vi "BioFeedback10(SaveStabilityData).vi"(0 "UI Data Right":path=path "C:/Users/Tinggroup/Desktop/VRMuscleActivationVisualizer/VRBiofeedback_v2/assets/RightEMGData.txt", 7 "Frames Per Second":dbl=30.0, 9 "Start Trial":bool, 11 "End Trial":bool, 12 "Data Directory":path, 13 "File Name":string, 14 "Extension":string="_EMG.txt") -> ()   [LabVIEW 2016]
uses:
  <vilib>/Utility/error.llb/DialogType.ctl
  <vilib>/Analysis/5stat.llb/RMS (DBL).vi
  <vilib>/Waveform/WDTOps.llb/WDT Append Waveforms DBL.vi
  <vilib>/Waveform/WDTFileIO.llb/Export Waveforms To Spreadsheet File (1D).vi
  <vilib>/Analysis/NI_AALPro.lvlib
panel:
  out "ReturnData":dbl[](array[numeric])
  in  "StdDevIndex":dbl=3.0
  in  "MeanIndex":dbl=2.0
  in  "MaxIndex":dbl=1.0
  in  "MinIndex":dbl
  out "Stability Data":dbl[][](array[numeric])
  out "2d target":cluster{dbl[], dbl[]}[](graph)
  out "trialFilteredData":waveform(dbl)[](array[waveform])
  out "filteredWaveforms":waveform(dbl)[](array[waveform])
  in  "UI Ampl Error Path":path=path "C:/Users/Tinggroup/Desktop/VRMuscleActivationVisualizer/VRBiofeedback_v2/assets/BiofeedbackAmplitudeError.txt"
  in  "UI L/R Error Path":path=path "C:/Users/Tinggroup/Desktop/VRMuscleActivationVisualizer/VRBiofeedback_v2/assets/BiofeedbackLRError.txt"
  out "LeftPercentActivation":dbl
  out "RightPercentActivation":dbl
  out "LeftMovingAvg":dbl
  out "RightMovingAvg":dbl
  in  "AutoAnalyzeStablity":bool
  out "RMS Left Single Bucket":dbl(graph)
  out "PointCluster":cluster{dbl[], dbl[]}
  out "combined y value":dbl
  out "Acquiring Max":bool
  in  "endGetMax":bool
  in  "startGetMax":bool
  in  "Right Max":dbl
  in  "Left Max":dbl
  in  "Amplitude Error":dbl
  in  "L/R error":dbl
  in  "RightSignalB":dbl=6.0
  in  "RightSignalA":dbl=5.0
  in  "LefftSignalB":dbl=2.0
  in  "LeftSignalA":dbl=1.0
  out "Aggregate 8":waveform(dbl)[](array[waveform])
  in  "UI Data Left":path=path "C:/Users/Tinggroup/Desktop/VRMuscleActivationVisualizer/VRBiofeedback_v2/assets/LeftEMGData.txt"
  in  "EMG Input Device\nProduct Type":string="USB-6009"
  out "DispLeftMovingAvg":dbl(slide) caption="Left" max=1.0 scale=0.0..100.0
  out "DispRightMovingAvg":dbl(slide) caption="Right" max=0.01 scale=0.0..100.0
  out "RMS Right":dbl(graph)
  out "RMS Left":dbl(graph)
  out "RMS 8":dbl(graph)
  out "RMS 7":dbl(graph)
  out "RMS 6":dbl(graph)
  out "RMS 5":dbl(graph)
  out "RMS 4":dbl(graph)
  out "RMS 3":dbl(graph)
  out "RMS 2":dbl(graph)
  out "RMS 1":dbl(graph)
  out "Aggregate7":waveform(dbl)[](array[waveform])
  out "Aggregate6":waveform(dbl)[](array[waveform])
  out "Aggregate5":waveform(dbl)[](array[waveform])
  out "Aggregate4":waveform(dbl)[](array[waveform])
  out "Aggregate3":waveform(dbl)[](array[waveform])
  out "Aggregate2":waveform(dbl)[](array[waveform])
  out "Aggregate1":waveform(dbl)[](array[waveform])
  out "Wfm8":waveform(dbl)(graph)
  out "Wfm7":waveform(dbl)(graph)
  out "Wfm6":waveform(dbl)(graph)
  out "Wfm5":waveform(dbl)(graph)
  out "Wfm4":waveform(dbl)(graph)
  out "Wfm3":waveform(dbl)(graph)
  out "Wfm2":waveform(dbl)(graph)
  out "Wfm1":waveform(dbl)(graph)
  out "Trial Raw Waveforms":waveform(dbl)[](graph)
  in  "UI Percent Path":path=path "C:/Users/Tinggroup/Desktop/VRMuscleActivationVisualizer/VRBiofeedback_v2/assets/BiofeedbackTargetPercentage.txt"
  in  "Target Percentage":dbl=10.0
  out "Trial In Progress":bool
  in  "Lower Cut-Off":dbl=20.0
  in  "Upper Cut-Off":dbl=300.0
  out "raw data":dynamicdata(graph)
  out "Bufffer Index":dbl
  out "Frames in Buffer":dbl
  out "Samples per frame":dbl
  out "Reset Data Acquisition\nAnd UI Updating":bool=TRUE
  in  "Moving Average Length (s)":dbl=0.5
  in  "Sample rate (Hz)":dbl=2000.0
  in  "End Program":bool
  # "Saving Trial Data"
  # "Set Target and Box Size"
  # "Set Scale"
  # "These scale the thermometers and are used in mean calculation"
  # "Analyze Stability of Displayed Data"
  # "Auto Analyze Stability begins calculating stability\nAs soon as dot enters the target zone and stops \nonce the dot leaves the target zone (Not Yet Implemented)"
  # "Channels used in Display"
  # "Filter and Process Parameters"
  # "Dimension1 - Signal\nDimension2 - property"
  # "Min"
  # "Max"
  # "Mean"
  # "StdDev"
  # "Changes are made instantly and cause moving average to reset to zero"
  # "for testing smaller sample\nsizes in getting max/min\nand stability data"
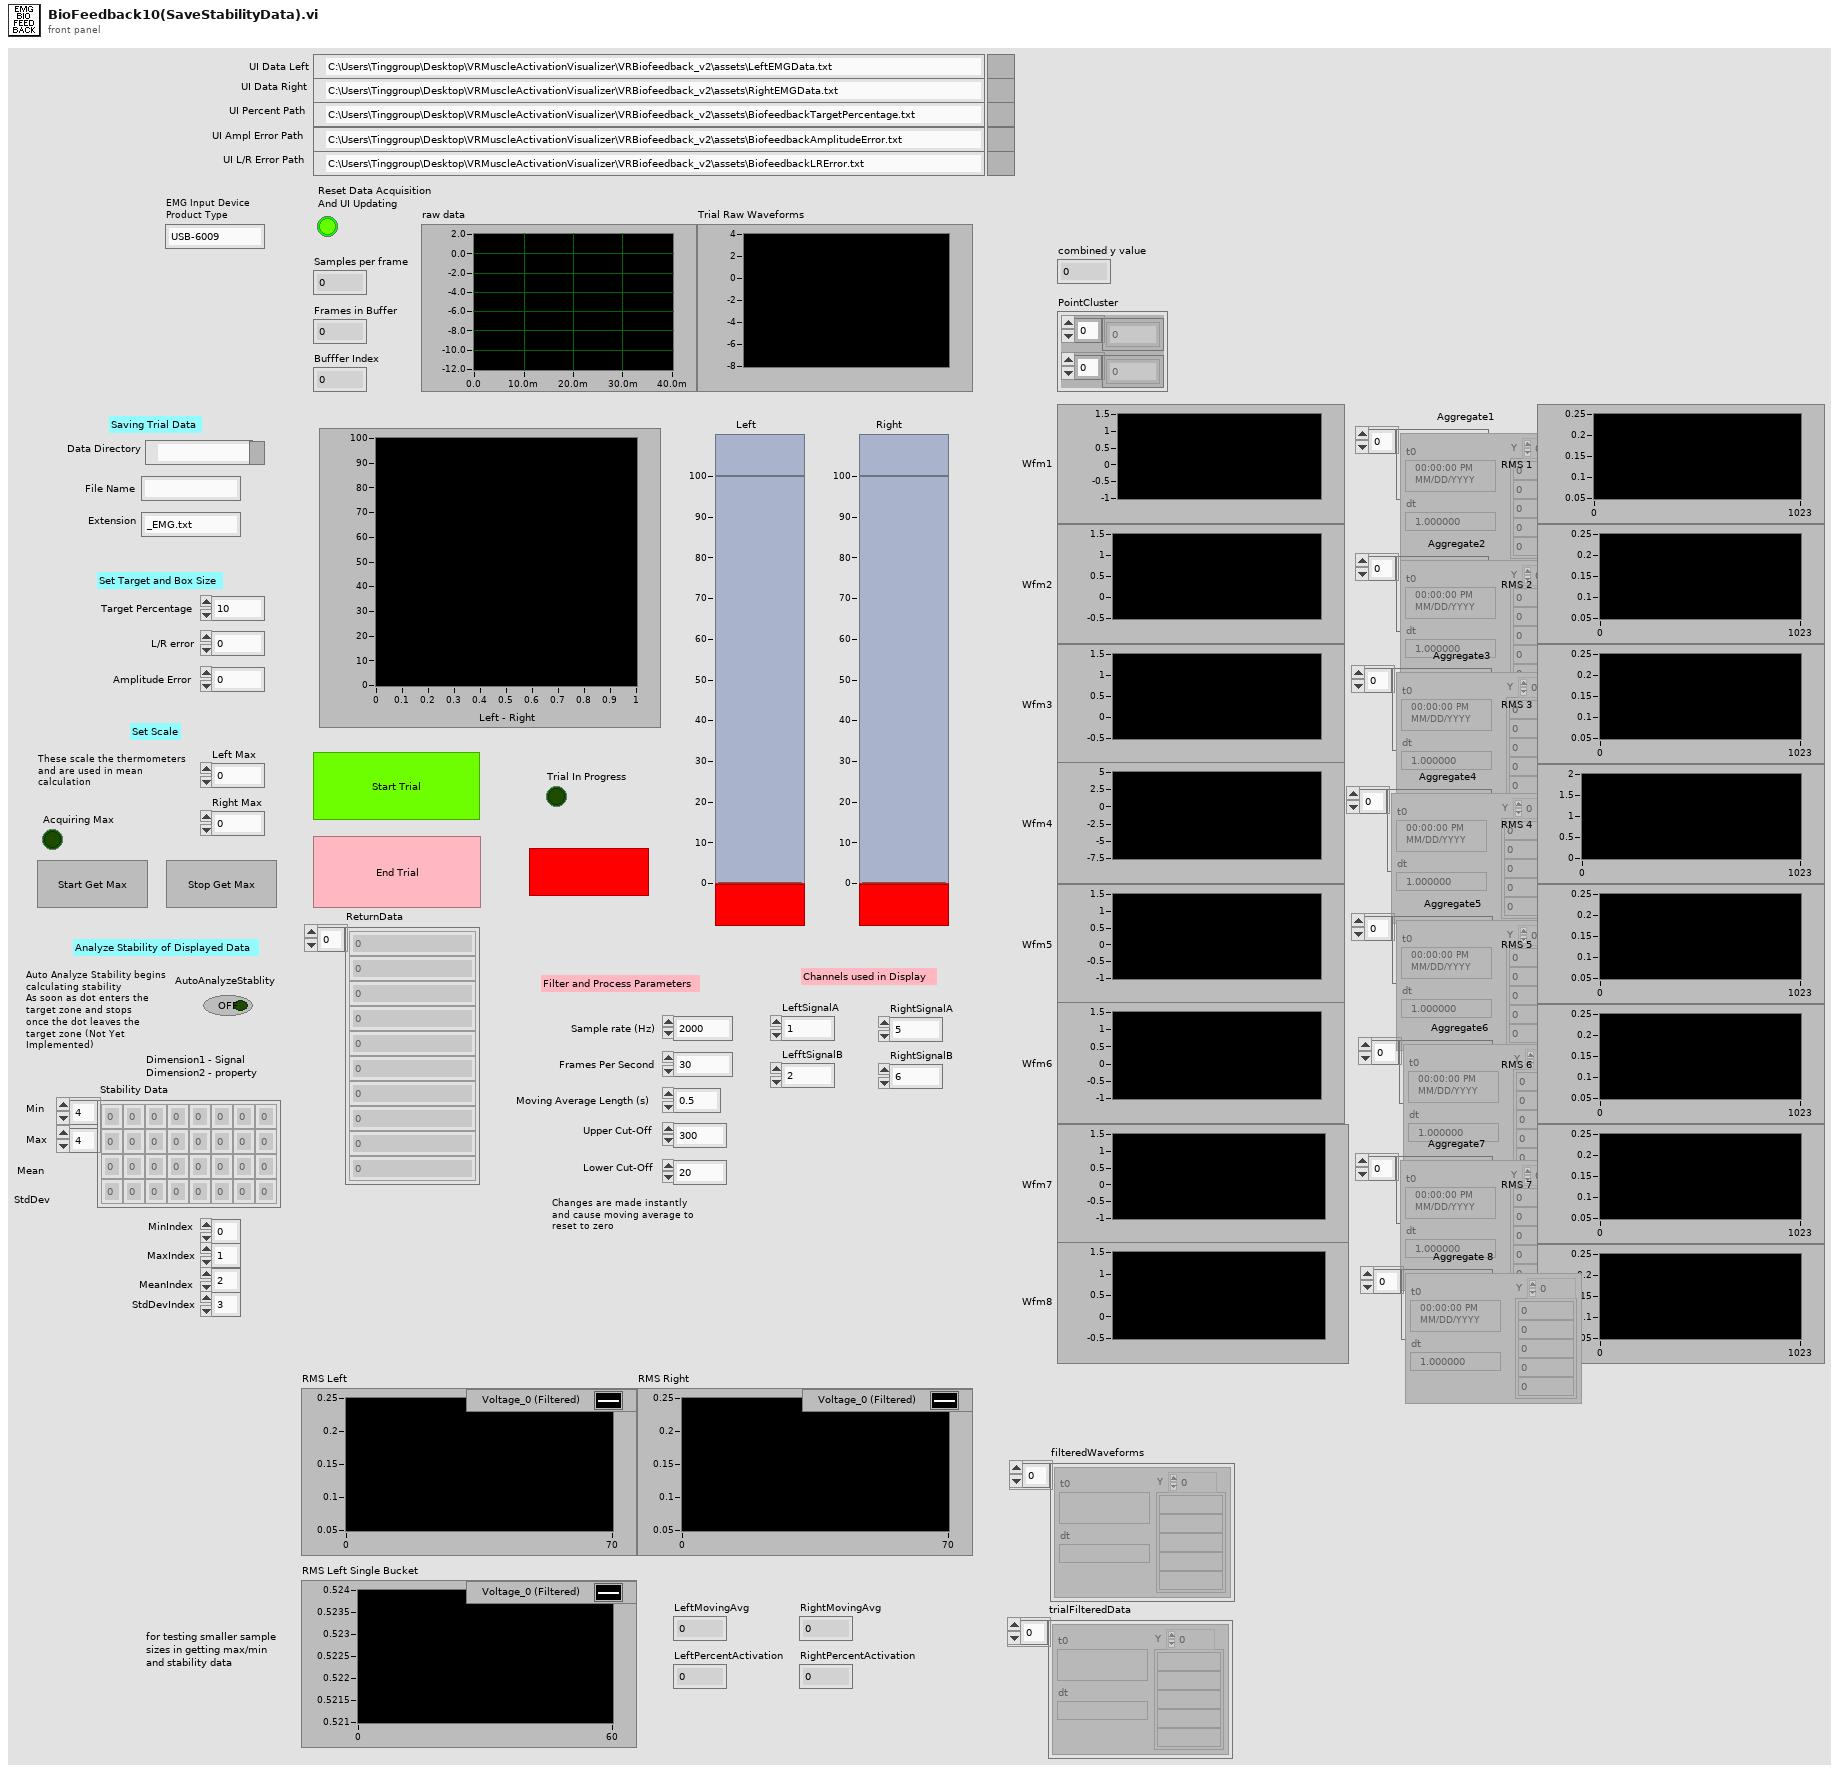
[diagram p1: front panel]
types:
  T1 = typedef "DialogType.ctl" = u16
  T2 = typedef "WaveformArrayControl.ctl" = waveform(dbl)[]
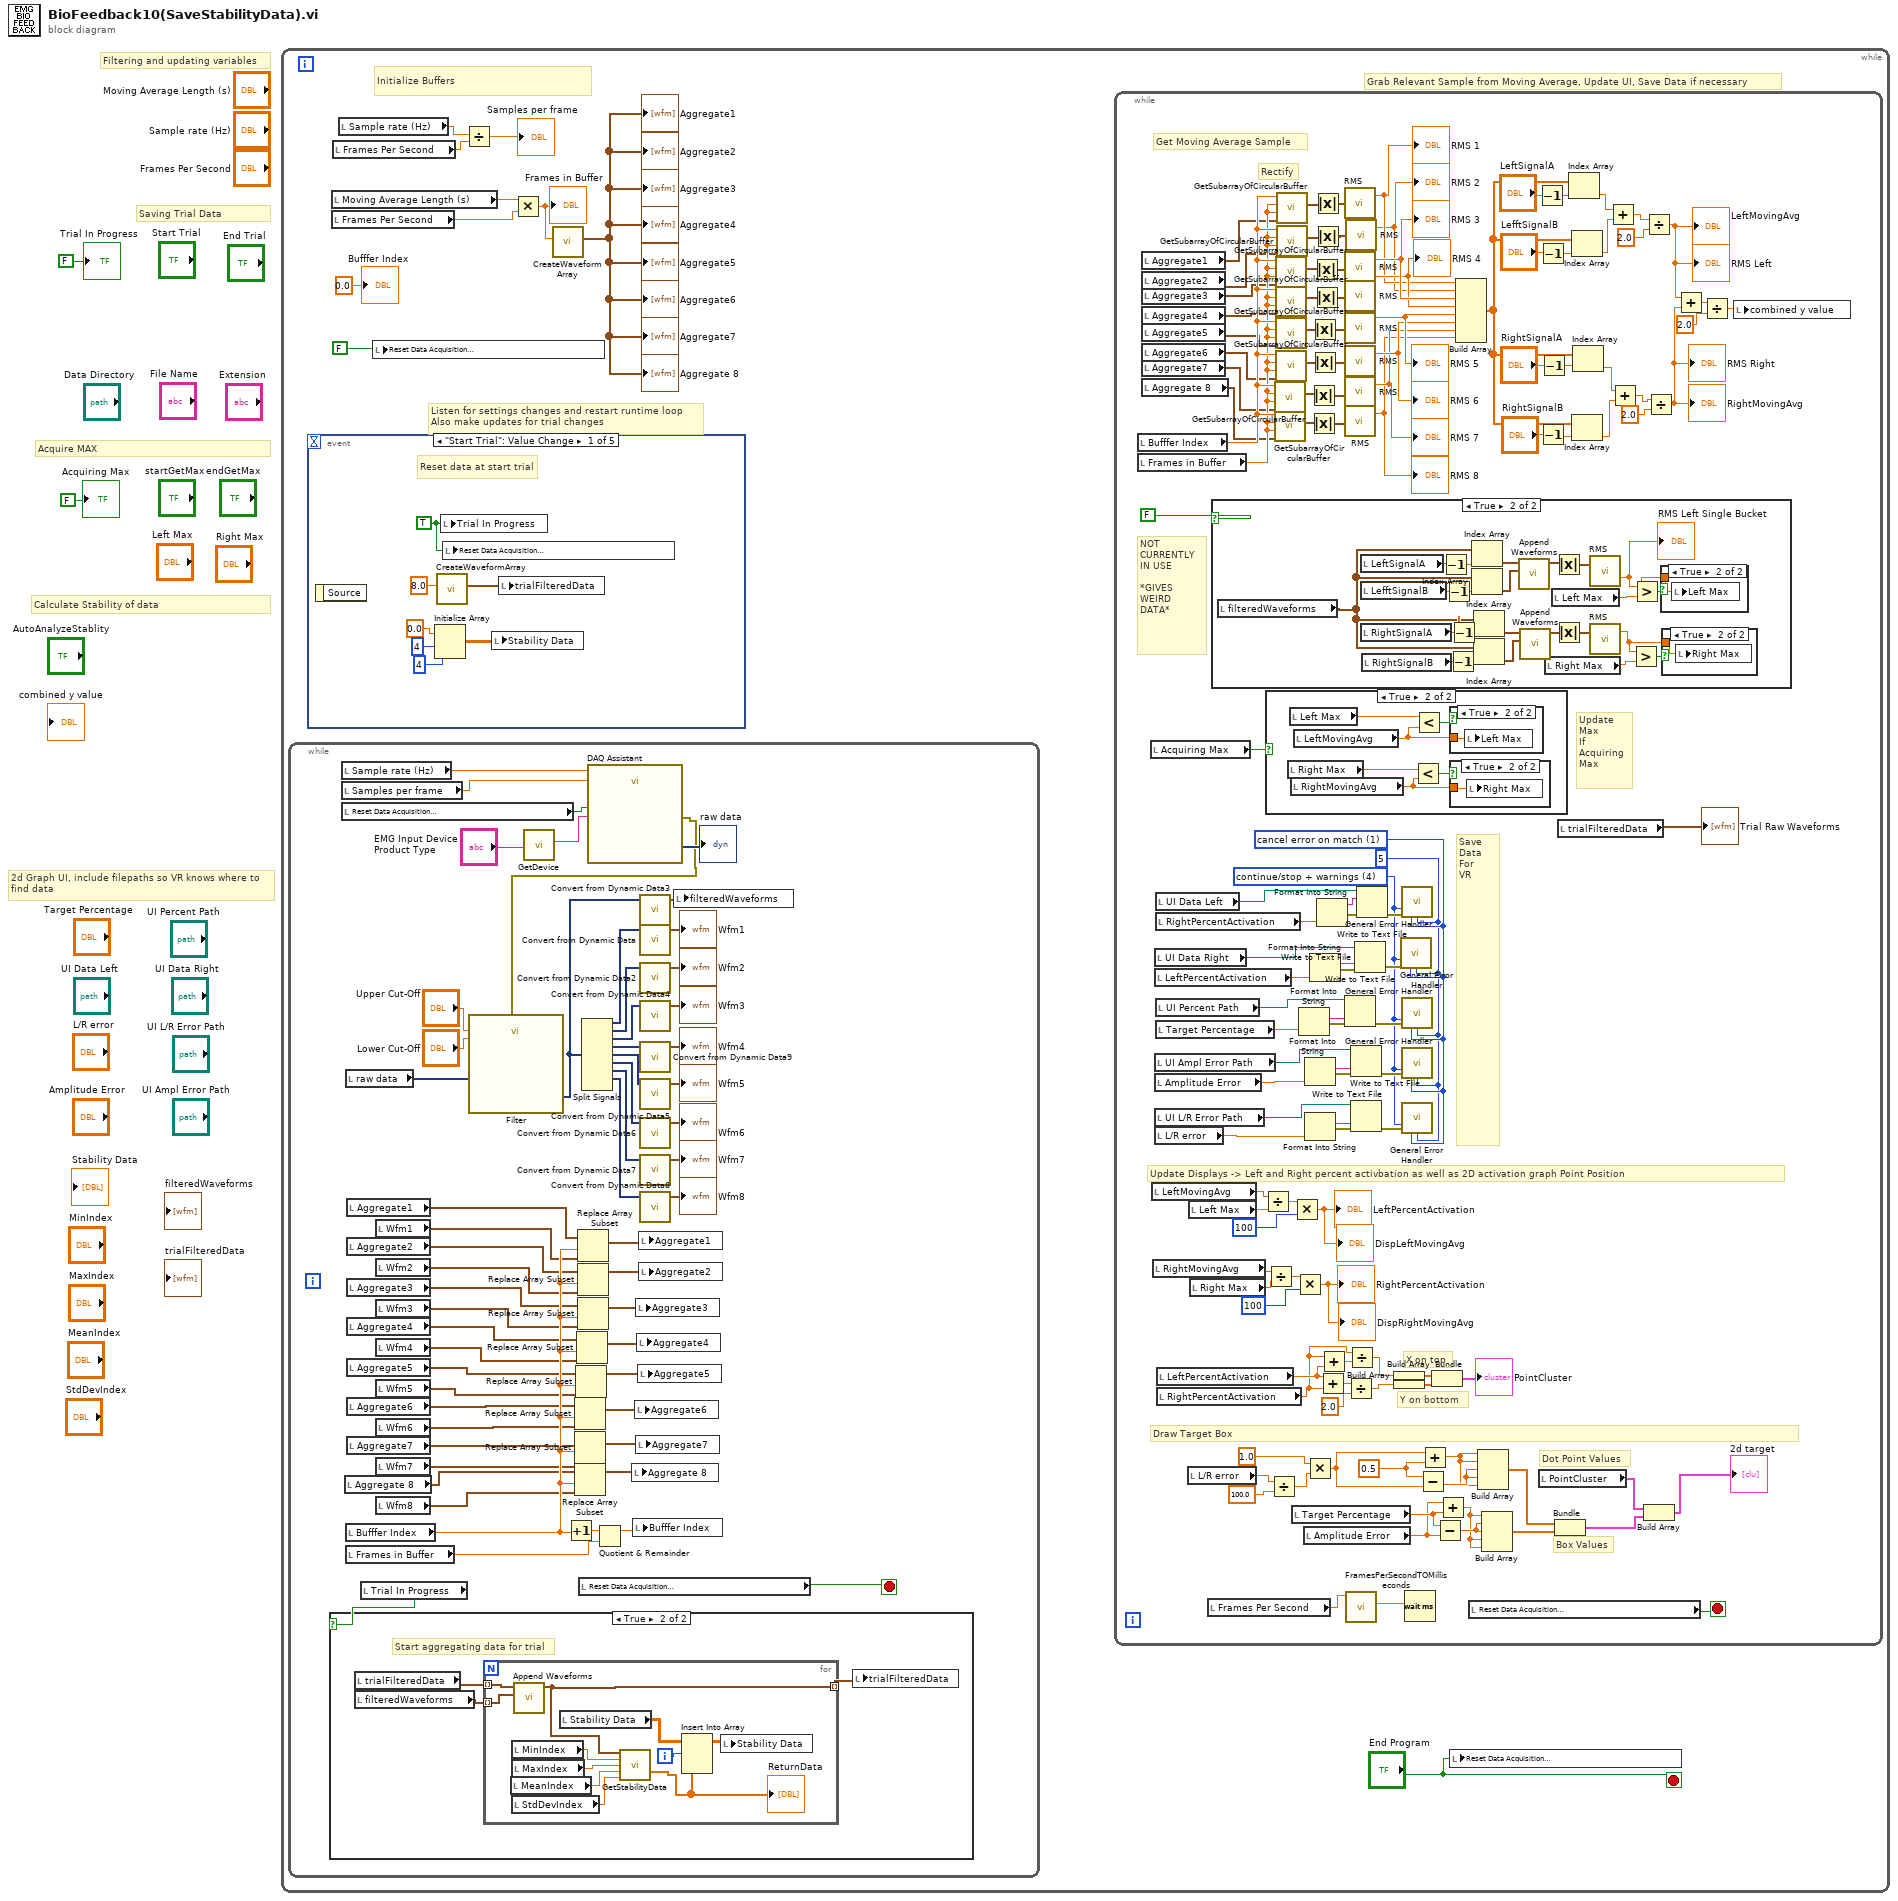
[diagram p0: block diagram]
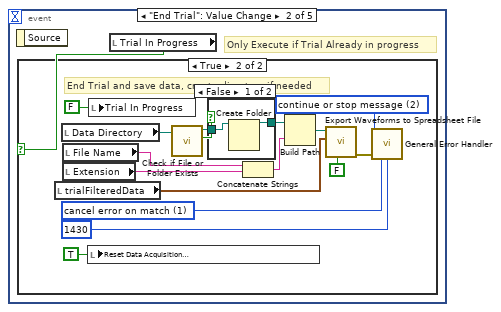
[diagram p2: hidden frame]
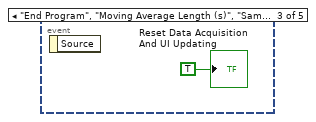
[diagram p5: hidden frame]
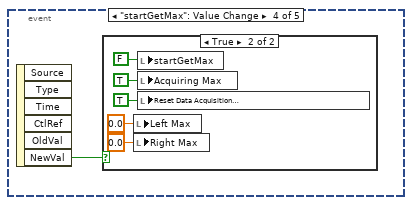
[diagram p6: hidden frame]
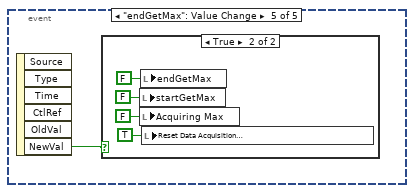
[diagram p8: hidden frame]
diagram:
  # "Calculate Stability of data"
  # "Acquire MAX"
  # "Filtering and updating variables"
  # "Saving Trial Data"
  # "2d Graph UI, include filepaths so VR knows where to find data"
  n1 = while {
    stop <- "End Program" stop-if-true
    # "Grab Relevant Sample from Moving Average, Update UI, Save Data if necessary"
    # "Initialize Buffers"
    # "Listen for settings changes and restart runtime loop\nAlso make updates for trial changes"
    n2 = while {
      stop <- w262 stop-if-true
      n3 = local read "Sample rate (Hz)"() -> (w269:dbl)
      n4 = local read "Samples per frame"() -> (w268:dbl)
      n5 = local read "Reset Data Acquisition\nAnd UI Updating"() -> (w261:bool)
      n6 = local read "Aggregate 8"() -> (w218:waveform(dbl)[])
      n7 = local read "raw data"() -> (w267:dynamicdata)
      n8 = local read "Bufffer Index"() -> (w243:dbl)
      n9 = local read "Frames in Buffer"() -> (w264:dbl)
      n10 = local read "Aggregate1"() -> (w242:waveform(dbl)[])
      n11 = local read "Aggregate2"() -> (w240:waveform(dbl)[])
      n12 = local read "Aggregate3"() -> (w238:waveform(dbl)[])
      n13 = local read "Aggregate4"() -> (w236:waveform(dbl)[])
      n14 = local read "Aggregate5"() -> (w234:waveform(dbl)[])
      n15 = local read "Aggregate6"() -> (w232:waveform(dbl)[])
      n16 = local read "Aggregate7"() -> (w230:waveform(dbl)[])
      n17 = local read "Trial In Progress"() -> (w220:bool)
      n18 = case shown="True" w220 {
        frame False {
        }
        frame True {
          # "Start aggregating data for trial"
          n19 = local read "trialFilteredData"() -> (w271:waveform(dbl)[])
          n20 = local read "filteredWaveforms"() -> (w272:waveform(dbl)[])
          n21 = for {
            tunnel: w272 -> [w282] mode=indexing
            tunnel: w271 -> [w283] mode=indexing
            tunnel: [w274] -> w270 mode=indexing
            i -> [w275]
            n22 = local read "MeanIndex"() -> (w278:dbl)
            n23 = local read "MinIndex"() -> (w276:dbl)
            n24 = local read "MaxIndex"() -> (w277:dbl)
            n25 = local read "StdDevIndex"() -> (w279:dbl)
            n26 = call-poly <vilib>:"Append Waveforms.vi"("waveform B"=w282, "waveform A"=w283) -> ("waveform out"=w274:waveform(dbl))  [unwired: 8 in, 1 out]
            n27 = local read "Stability Data"() -> (w280:dbl[][])
            n28 = call "GetStabilityData.vi"("ProvidedData"=w274, "MinIndex"=w276, "MaxIndex"=w277, "MeanIndex"=w278, "StdDevIndex"=w279) -> ("ReturnData"=w273:dbl[])  [unwired: 10 in]
            "ReturnData" <- w273
            n29 = Insert Into Array(array=w280, index (row)=w275, new element=w273) -> (w281:dbl[][])  [unwired: 1 in]
            n30 = local write "Stability Data"(w281) -> ()
          }
          n31 = local write "trialFilteredData"(w270) -> ()
        }
      }
      n32 = local read "Wfm1"() -> (w241:waveform(dbl))
      n33 = local read "Wfm2"() -> (w239:waveform(dbl))
      n34 = local read "Wfm3"() -> (w237:waveform(dbl))
      n35 = local read "Wfm4"() -> (w235:waveform(dbl))
      n36 = local read "Wfm5"() -> (w233:waveform(dbl))
      n37 = local read "Wfm6"() -> (w231:waveform(dbl))
      n38 = local read "Wfm7"() -> (w229:waveform(dbl))
      n39 = local read "Wfm8"() -> (w228:waveform(dbl))
      n40 = call "GetDevice.vi"("EMG Input Device\nProduct Type"="EMG Input Device\nProduct Type") -> ("DAQmx Device Name"=w216:tag)  [unwired: 10 in]
      n41 = Increment(x=w243) -> (x+1=w263:dbl)
      n42 = Replace Array Subset(array=w232, new element=w231, index=w243) -> (w222:waveform(dbl)[])
      n43 = Replace Array Subset(array=w230, new element=w229, index=w243) -> (w221:waveform(dbl)[])
      n44 = Replace Array Subset(array=w218, new element=w228, index=w243) -> (w219:waveform(dbl)[])
      n45 = Replace Array Subset(array=w234, new element=w233, index=w243) -> (w223:waveform(dbl)[])
      n46 = Replace Array Subset(array=w236, new element=w235, index=w243) -> (w224:waveform(dbl)[])
      n47 = Replace Array Subset(array=w242, new element=w241, index=w243) -> (w227:waveform(dbl)[])
      n48 = Replace Array Subset(array=w240, new element=w239, index=w243) -> (w226:waveform(dbl)[])
      n49 = Replace Array Subset(array=w238, new element=w237, index=w243) -> (w225:waveform(dbl)[])
      n50 = local read "Reset Data Acquisition\nAnd UI Updating"() -> (w262:bool)
      n51 = call "DAQ Assistant"("rate"=w269, "number of samples"=w268, "stop (T)"=w261, "device name"=w216) -> ("data"=→"raw data":dynamicdata, "error out"=w213:errorcluster)  [unwired: 13 in, 1 out]
      n52 = call "Filter"("error in (no error)"=w213, "Lower Cut-Off"="Lower Cut-Off", "Upper Cut-Off"="Upper Cut-Off", "Signal"=w267) -> ("Filtered Signal"=w212:dynamicdata)  [unwired: 6 in, 1 out]
      n53 = Split Signals(w212) -> (w259:dynamicdata, w258:dynamicdata, w257:dynamicdata, w256:dynamicdata, w255:dynamicdata, w254:dynamicdata, w253:dynamicdata, w252:dynamicdata)  [unwired: 9 in, 1 out]
      n54 = Quotient & Remainder(x=w263, y=w264) -> (x-y*floor(x/y)=w265:dbl)  [unwired: 1 out]
      n55 = local write "Aggregate 8"(w219) -> ()
      n56 = local write "Bufffer Index"(w265) -> ()
      n57 = local write "Aggregate6"(w222) -> ()
      n58 = local write "Aggregate3"(w225) -> ()
      n59 = local write "Aggregate7"(w221) -> ()
      n60 = local write "Aggregate4"(w224) -> ()
      n61 = local write "Aggregate5"(w223) -> ()
      n62 = local write "Aggregate1"(w227) -> ()
      n63 = local write "Aggregate2"(w226) -> ()
      n64 = call "Convert from Dynamic Data3"("Dynamic Data Type"=w212) -> ("Array of Waveform"=w214:waveform(dbl)[])  [unwired: 3 in]
      n65 = call "Convert from Dynamic Data"("Dynamic Data Type"=w259) -> ("Waveform"=→"Wfm1":waveform(dbl))  [unwired: 3 in]
      n66 = call "Convert from Dynamic Data2"("Dynamic Data Type"=w258) -> ("Waveform"=→"Wfm2":waveform(dbl))  [unwired: 3 in]
      n67 = call "Convert from Dynamic Data4"("Dynamic Data Type"=w257) -> ("Waveform"=→"Wfm3":waveform(dbl))  [unwired: 3 in]
      n68 = call "Convert from Dynamic Data9"("Dynamic Data Type"=w256) -> ("Waveform"=→"Wfm4":waveform(dbl))  [unwired: 3 in]
      n69 = call "Convert from Dynamic Data5"("Dynamic Data Type"=w255) -> ("Waveform"=→"Wfm5":waveform(dbl))  [unwired: 3 in]
      n70 = call "Convert from Dynamic Data6"("Dynamic Data Type"=w254) -> ("Waveform"=→"Wfm6":waveform(dbl))  [unwired: 3 in]
      n71 = call "Convert from Dynamic Data7"("Dynamic Data Type"=w253) -> ("Waveform"=→"Wfm7":waveform(dbl))  [unwired: 3 in]
      n72 = call "Convert from Dynamic Data8"("Dynamic Data Type"=w252) -> ("Waveform"=→"Wfm8":waveform(dbl))  [unwired: 3 in]
      n73 = local write "filteredWaveforms"(w214) -> ()
    }
    n74 = event shown="[0] \"Start Trial\": Value Change" {
      selector: _ -> [_ _ _ _ _]
      dyn-events: _ -> [_ _ _ _ _]
      timeout: _ -> [_ _ _ _ _]
      event "Start Trial": Value Change {
        w19 = TRUE ("Trial In Progress")
        # "Reset data at start trial"
        n75 = event-data() -> ()  [unwired: 1 in, 1 out]
        n76 = Initialize Array(0.0 ("element"), 4 ("dimension size"), 4 ("dimension size")) -> (w13:dbl[][])
        n77 = call "CreateWaveformArray.vi"("bufferSize"=8.0) -> ("initialized array"=w18:waveform(dbl)[])  [unwired: 5 in, 1 out]
        n78 = local write "Trial In Progress"(w19) -> ()
        n79 = local write "Reset Data Acquisition\nAnd UI Updating"(w19) -> ()
        n80 = local write "Stability Data"(w13) -> ()
        n81 = local write "trialFilteredData"(w18) -> ()
      }
      event "End Trial": Value Change {
        # "Only Execute if Trial Already in progress"
        n82 = event-data() -> ()  [unwired: 1 in, 1 out]
        n83 = local read "Trial In Progress"() -> (w20:bool)
        n84 = case shown="True" w20 {
          frame False {
          }
          frame True {
            w29 = T1 2 items=["no dialog", "OK message", "continue or stop message", "OK message + warnings", "continue/stop + warnings"] ("type of dialog (OK msg:1)")
            w30 = 1 items=["no exception", "cancel error on match", "set error on match"] ("[exception action] (none:0)")
            # "End Trial and save data, create directory if needed"
            n85 = local read "trialFilteredData"() -> (w22:waveform(dbl)[])
            n86 = local read "Data Directory"() -> (w32:path)
            n87 = local read "File Name"() -> (w24:string)
            n88 = local read "Extension"() -> (w25:string)
            n89 = local write "Reset Data Acquisition\nAnd UI Updating"(TRUE ("Reset Data Acquisition\nAnd UI Updating")) -> ()
            n90 = local write "Trial In Progress"(FALSE ("Trial In Progress")) -> ()
            n91 = call <vilib>:"Check if File or Folder Exists.vi"("path"=w32) -> ("file or folder exists?"=w34:bool, "dup path"=w33:path)  [unwired: 8 in, 1 out]
            n92 = case shown="False" w34 {
              tunnel: [w37 w39] -> w28
              tunnel: w33 -> [w38 w39]
              frame False {
                n93 = Create Folder(path (use dialog)=w38) -> (created path=w37:path)  [unwired: 2 in, 2 out]
              }
              frame True {
              }
            }
            n94 = Concatenate Strings(w24, w25) -> (w23:string)
            n95 = Build Path(base path=w28, name or relative path=w23) -> (appended path=w27:path)
            n96 = call-poly <vilib>:"Export Waveforms to Spreadsheet File.vi"("append to file? (new file:F)"=FALSE, "waveforms"=w22, "file path (dialog if empty)"=w27) -> ("error out"=w21:errorcluster)  [unwired: 7 in, 1 out]
            n97 = call <vilib>:"General Error Handler.vi"("type of dialog (OK msg:1)"=w29, "error in (no error)"=w21, "[exception action] (none:0)"=w30, "[exception code]"=1430) -> ()  [unwired: 7 in, 5 out]
          }
        }
      }
      event "End Program", "Moving Average Length (s)", "Sample rate (Hz)", "Frames Per Second": Value Change {
        n98 = event-data() -> ()  [unwired: 1 in, 1 out]
        "Reset Data Acquisition\nAnd UI Updating" <- TRUE
      }
      event "startGetMax": Value Change {
        n99 = event-data() -> ("NewVal"=w41:bool)  [unwired: 1 in, 5 out]
        n100 = case shown="True" w41 {
          frame False {
          }
          frame True {
            n101 = local write "Left Max"(0.0 ("Left Max")) -> ()
            n102 = local write "Right Max"(0.0 ("Right Max")) -> ()
            n103 = local write "startGetMax"(FALSE) -> ()
            n104 = local write "Acquiring Max"(TRUE ("Acquiring Max")) -> ()
            n105 = local write "Reset Data Acquisition\nAnd UI Updating"(TRUE ("Reset Data Acquisition\nAnd UI Updating")) -> ()
          }
        }
      }
      event "endGetMax": Value Change {
        n106 = event-data() -> ("NewVal"=w47:bool)  [unwired: 1 in, 5 out]
        n107 = case shown="True" w47 {
          frame False {
          }
          frame True {
            n108 = local write "startGetMax"(FALSE ("startGetMax")) -> ()
            n109 = local write "Acquiring Max"(FALSE ("Acquiring Max")) -> ()
            n110 = local write "endGetMax"(FALSE ("endGetMax")) -> ()
            n111 = local write "Reset Data Acquisition\nAnd UI Updating"(TRUE ("Reset Data Acquisition\nAnd UI Updating")) -> ()
          }
        }
      }
    }
    n112 = local read "Moving Average Length (s)"() -> (w9:dbl)
    n113 = local read "Frames Per Second"() -> (w8:dbl)
    n114 = local read "Frames Per Second"() -> (w11:dbl)
    n115 = local read "Sample rate (Hz)"() -> (w12:dbl)
    n116 = local write "Reset Data Acquisition\nAnd UI Updating"(FALSE) -> ()
    n117 = Divide(x=w12, y=w11) -> (x/y=→"Samples per frame":dbl)
    n118 = Multiply(x=w9, y=w8) -> (x*y=w5:dbl)
    "Frames in Buffer" <- w5
    n119 = call "CreateWaveformArray.vi"("bufferSize"=w5) -> ("initialized array"=→"Aggregate1" →"Aggregate2" →"Aggregate3" →"Aggregate4" →"Aggregate5" →"Aggregate6" →"Aggregate7" →"Aggregate 8":waveform(dbl)[])  [unwired: 5 in, 1 out]
    n120 = while {
      stop <- w178 stop-if-true
      w104 = 0.5 ("element")
      w57 = T1 4 items=["no dialog", "OK message", "continue or stop message", "OK message + warnings", "continue/stop + warnings"] ("type of dialog (OK msg:1)")
      w56 = 1 items=["no exception", "cancel error on match", "set error on match"] ("[exception action] (none:0)")
      w55 = 5 ("[exception code]")
      # "Y on bottom"
      # "X on top"
      # "Dot Point Values"
      # "Box Values"
      # "Update Displays -> Left and Right percent activbation as well as 2D activation graph Point Position"
      # "NOT\nCURRENTLY\nIN USE\n\n*GIVES\nWEIRD\nDATA*"
      # "Draw Target Box"
      # "Update\nMax\nIf \nAcquiring\nMax"
      # "Save\nData\nFor\nVR"
      # "Get Moving Average Sample"
      # "Rectify"
      n121 = local read "Bufffer Index"() -> (w169:dbl)
      n122 = local read "Frames in Buffer"() -> (w168:dbl)
      n123 = local read "Aggregate1"() -> (w167:waveform(dbl)[])
      n124 = local read "Aggregate2"() -> (w163:waveform(dbl)[])
      n125 = local read "Aggregate3"() -> (w166:waveform(dbl)[])
      n126 = local read "Aggregate4"() -> (w162:waveform(dbl)[])
      n127 = local read "Aggregate5"() -> (w165:waveform(dbl)[])
      n128 = local read "Aggregate6"() -> (w164:waveform(dbl)[])
      n129 = local read "Aggregate7"() -> (w161:waveform(dbl)[])
      n130 = local read "Aggregate 8"() -> (w135:waveform(dbl)[])
      n131 = local read "Acquiring Max"() -> (w90:bool)
      n132 = local read "LeftMovingAvg"() -> (w86:dbl)
      n133 = local read "RightMovingAvg"() -> (w82:dbl)
      n134 = local read "UI Data Right"() -> (w173:path)
      n135 = local read "LeftPercentActivation"() -> (w171:dbl)
      n136 = local read "UI Ampl Error Path"() -> (w58:path)
      n137 = local read "Amplitude Error"() -> (w59:dbl)
      n138 = local read "UI L/R Error Path"() -> (w61:path)
      n139 = local read "L/R error"() -> (w60:dbl)
      n140 = local read "UI Data Left"() -> (w143:path)
      n141 = local read "RightPercentActivation"() -> (w145:dbl)
      n142 = local read "UI Percent Path"() -> (w137:path)
      n143 = local read "Target Percentage"() -> (w136:dbl)
      n144 = local read "LeftPercentActivation"() -> (w75:dbl)
      n145 = local read "RightPercentActivation"() -> (w73:dbl)
      n146 = local read "L/R error"() -> (w115:dbl)
      n147 = local read "Left Max"() -> (w85:dbl)
      n148 = local read "Right Max"() -> (w81:dbl)
      n149 = local read "Frames Per Second"() -> (w177:dbl)
      n150 = case shown="True" FALSE {
        frame False {
        }
        frame True {
          n151 = local read "filteredWaveforms"() -> (w187:waveform(dbl)[])
          n152 = local read "LeftSignalA"() -> (w195:dbl)
          n153 = local read "LefftSignalB"() -> (w193:dbl)
          n154 = local read "RightSignalA"() -> (w191:dbl)
          n155 = local read "RightSignalB"() -> (w188:dbl)
          n156 = Decrement(x=w195) -> (x-1=w194:dbl)
          n157 = Decrement(x=w193) -> (x-1=w192:dbl)
          n158 = Decrement(x=w188) -> (x-1=w189:dbl)
          n159 = Decrement(x=w191) -> (x-1=w190:dbl)
          n160 = Index Array(array=w187, index=w194) -> (element=w196:waveform(dbl))
          n161 = Index Array(array=w187, index=w192) -> (element=w197:waveform(dbl))
          n162 = Index Array(array=w187, index=w190) -> (element=w208:waveform(dbl))
          n163 = Index Array(array=w187, index=w189) -> (element=w207:waveform(dbl))
          n164 = call-poly <vilib>:"Append Waveforms.vi"("waveform B"=w197, "waveform A"=w196) -> ("waveform out"=w203:waveform(dbl))  [unwired: 8 in, 1 out]
          n165 = call-poly <vilib>:"Append Waveforms.vi"("waveform B"=w207, "waveform A"=w208) -> ("waveform out"=w206:waveform(dbl))  [unwired: 8 in, 1 out]
          n166 = local read "Right Max"() -> (w202:dbl)
          n167 = local read "Left Max"() -> (w209:dbl)
          n168 = Absolute Value(x=w203) -> (abs(x)=w204:waveform(dbl))
          n169 = Absolute Value(x=w206) -> (abs(x)=w205:waveform(dbl))
          n170 = call-poly <vilib>:"RMS.vi"("X"=w204) -> ("rms value"=w198:dbl)  [unwired: 1 out]
          "RMS Left Single Bucket" <- w198
          n171 = call-poly <vilib>:"RMS.vi"("X"=w205) -> ("rms value"=w201:dbl)  [unwired: 1 out]
          n172 = Greater?(x=w201, y=w202) -> (0:w200:bool)
          n173 = Greater?(x=w198, y=w209) -> (0:w199:bool)
          n174 = case shown="True" w199 {
            tunnel: w198 -> [_ w211]
            frame False {
            }
            frame True {
              n175 = local write "Left Max"(w211) -> ()
            }
          }
          n176 = case shown="True" w200 {
            tunnel: w201 -> [_ w210]
            frame False {
            }
            frame True {
              n177 = local write "Right Max"(w210) -> ()
            }
          }
        }
      }
      n178 = Divide(x=w86, y=w85) -> (x/y=w87:dbl)
      n179 = case shown="True" w90 {
        frame False {
        }
        frame True {
          n180 = local read "Right Max"() -> (w181:dbl)
          n181 = local read "Left Max"() -> (w184:dbl)
          n182 = local read "RightMovingAvg"() -> (w179:dbl)
          n183 = local read "LeftMovingAvg"() -> (w183:dbl)
          n184 = Less?(x=w181, y=w179) -> (x < y?=w180:bool)
          n185 = Less?(x=w184, y=w183) -> (x < y?=w182:bool)
          n186 = case shown="True" w182 {
            tunnel: w183 -> [_ w186]
            frame False {
            }
            frame True {
              n187 = local write "Left Max"(w186) -> ()
            }
          }
          n188 = case shown="True" w180 {
            tunnel: w179 -> [_ w185]
            frame False {
            }
            frame True {
              n189 = local write "Right Max"(w185) -> ()
            }
          }
        }
      }
      n190 = Divide(x=w82, y=w81) -> (x/y=w83:dbl)
      n191 = Divide(x=w115, y=100.0) -> (x/y=w109:dbl)
      n192 = call "GetSubarrayOfCircularBuffer.vi"("initialized array"=w161, "buffer size"=w168, "subset size"=w168, "start index"=w169) -> ("initialized array 2"=w154:T2)  [unwired: 7 in]
      n193 = call "GetSubarrayOfCircularBuffer.vi"("initialized array"=w135, "buffer size"=w168, "subset size"=w168, "start index"=w169) -> ("initialized array 2"=w153:T2)  [unwired: 7 in]
      n194 = call "GetSubarrayOfCircularBuffer.vi"("initialized array"=w166, "buffer size"=w168, "subset size"=w168, "start index"=w169) -> ("initialized array 2"=w158:T2)  [unwired: 7 in]
      n195 = call "GetSubarrayOfCircularBuffer.vi"("initialized array"=w162, "buffer size"=w168, "subset size"=w168, "start index"=w169) -> ("initialized array 2"=w157:T2)  [unwired: 7 in]
      n196 = call "GetSubarrayOfCircularBuffer.vi"("initialized array"=w165, "buffer size"=w168, "subset size"=w168, "start index"=w169) -> ("initialized array 2"=w156:T2)  [unwired: 7 in]
      n197 = call "GetSubarrayOfCircularBuffer.vi"("initialized array"=w164, "buffer size"=w168, "subset size"=w168, "start index"=w169) -> ("initialized array 2"=w155:T2)  [unwired: 7 in]
      n198 = call "GetSubarrayOfCircularBuffer.vi"("initialized array"=w167, "buffer size"=w168, "subset size"=w168, "start index"=w169) -> ("initialized array 2"=w160:T2)  [unwired: 7 in]
      n199 = call "GetSubarrayOfCircularBuffer.vi"("initialized array"=w163, "buffer size"=w168, "subset size"=w168, "start index"=w169) -> ("initialized array 2"=w159:T2)  [unwired: 7 in]
      n200 = Multiply(x=w87, y=100) -> (x*y=→"DispLeftMovingAvg" →"LeftPercentActivation":dbl)
      n201 = local read "Target Percentage"() -> (w54:dbl)
      n202 = Multiply(x=w83, y=100) -> (x*y=→"DispRightMovingAvg" →"RightPercentActivation":dbl)
      n203 = Format Into String(w136) -> (resulting string=w138:string, error out=w139:errorcluster)  [unwired: 3 in]
      n204 = local read "Amplitude Error"() -> (w53:dbl)
      n205 = Format Into String(w59) -> (resulting string=w65:string, error out=w66:errorcluster)  [unwired: 3 in]
      n206 = Format Into String(w60) -> (resulting string=w62:string, error out=w63:errorcluster)  [unwired: 3 in]
      n207 = Multiply(x=1.0, y=w109) -> (x*y=w108:dbl)
      n208 = Absolute Value(x=w154) -> (abs(x)=w147:T2)
      n209 = Absolute Value(x=w153) -> (abs(x)=w146:T2)
      n210 = Absolute Value(x=w156) -> (abs(x)=w149:T2)
      n211 = Absolute Value(x=w155) -> (abs(x)=w148:T2)
      n212 = Format Into String(w171) -> (resulting string=w172:string, error out=w174:errorcluster)  [unwired: 3 in]
      n213 = Absolute Value(x=w158) -> (abs(x)=w151:T2)
      n214 = Absolute Value(x=w157) -> (abs(x)=w150:T2)
      n215 = Absolute Value(x=w160) -> (abs(x)=w152:T2)
      n216 = Absolute Value(x=w159) -> (abs(x)=w134:T2)
      n217 = Format Into String(w145) -> (resulting string=w142:string, error out=w144:errorcluster)  [unwired: 3 in]
      n218 = Add(x=w75, y=w73) -> (x+y=w77:dbl)
      n219 = Add(x=w73, y=w75) -> (x+y=w74:dbl)
      n220 = call-poly <vilib>:"RMS.vi"("X"=w152) -> ("rms value"=w128:dbl)  [unwired: 1 out]
      "RMS 1" <- w128
      n221 = call-poly <vilib>:"RMS.vi"("X"=w151) -> ("rms value"=w133:dbl)  [unwired: 1 out]
      "RMS 3" <- w133
      n222 = call-poly <vilib>:"RMS.vi"("X"=w150) -> ("rms value"=w132:dbl)  [unwired: 1 out]
      "RMS 4" <- w132
      n223 = call-poly <vilib>:"RMS.vi"("X"=w149) -> ("rms value"=w131:dbl)  [unwired: 1 out]
      "RMS 5" <- w131
      n224 = call-poly <vilib>:"RMS.vi"("X"=w148) -> ("rms value"=w130:dbl)  [unwired: 1 out]
      "RMS 6" <- w130
      n225 = call-poly <vilib>:"RMS.vi"("X"=w147) -> ("rms value"=w129:dbl)  [unwired: 1 out]
      "RMS 7" <- w129
      n226 = call-poly <vilib>:"RMS.vi"("X"=w146) -> ("rms value"=w126:dbl)  [unwired: 1 out]
      "RMS 8" <- w126
      n227 = Write to Text File(file (use dialog)=w137, text=w138, error in=w139) -> (error out=w140:errorcluster)  [unwired: 1 in, 2 out]
      n228 = call-poly <vilib>:"RMS.vi"("X"=w134) -> ("rms value"=w127:dbl)  [unwired: 1 out]
      "RMS 2" <- w127
      n229 = Divide(x=w77, y=2.0) -> (x/y=w76:dbl)
      n230 = call "FramesPerSecondTOMilliseconds.vi"("Thermometer\nFps"=w177) -> ("x*y"=w176:dbl)  [unwired: 10 in]
      n231 = Divide(x=w73, y=w74) -> (x/y=w72:dbl)
      n232 = Write to Text File(file (use dialog)=w58, text=w65, error in=w66) -> (error out=w67:errorcluster)  [unwired: 1 in, 2 out]
      n233 = Write to Text File(file (use dialog)=w61, text=w62, error in=w63) -> (error out=w64:errorcluster)  [unwired: 1 in, 2 out]
      n234 = Write to Text File(file (use dialog)=w173, text=w172, error in=w174) -> (error out=w175:errorcluster)  [unwired: 1 in, 2 out]
      n235 = Write to Text File(file (use dialog)=w143, text=w142, error in=w144) -> (error out=w141:errorcluster)  [unwired: 1 in, 2 out]
      n236 = Build Array(w72) -> (w120:dbl[])
      n237 = Build Array(w76) -> (w118:dbl[])
      n238 = call <vilib>:"General Error Handler.vi"("type of dialog (OK msg:1)"=w57, "error in (no error)"=w175, "[exception action] (none:0)"=w56, "[exception code]"=w55) -> ()  [unwired: 7 in, 5 out]
      n239 = call <vilib>:"General Error Handler.vi"("type of dialog (OK msg:1)"=w57, "error in (no error)"=w141, "[exception action] (none:0)"=w56, "[exception code]"=w55) -> ()  [unwired: 7 in, 5 out]
      n240 = call <vilib>:"General Error Handler.vi"("type of dialog (OK msg:1)"=w57, "error in (no error)"=w140, "[exception action] (none:0)"=w56, "[exception code]"=w55) -> ()  [unwired: 7 in, 5 out]
      n241 = call <vilib>:"General Error Handler.vi"("type of dialog (OK msg:1)"=w57, "error in (no error)"=w67, "[exception action] (none:0)"=w56, "[exception code]"=w55) -> ()  [unwired: 7 in, 5 out]
      n242 = call <vilib>:"General Error Handler.vi"("type of dialog (OK msg:1)"=w57, "error in (no error)"=w64, "[exception action] (none:0)"=w56, "[exception code]"=w55) -> ()  [unwired: 7 in, 5 out]
      n243 = Wait (ms)(milliseconds to wait=w176) -> ()  [unwired: 1 out]
      n244 = Subtract(x=w104, y=w108) -> (x-y=w114:dbl)
      n245 = Add(x=w108, y=w104) -> (x+y=w110:dbl)
      n246 = Bundle(w120, w118) -> (→"PointCluster":cluster{dbl[], dbl[]})  [unwired: 1 in]
      n247 = Subtract(x=w54, y=w53) -> (x-y=w112:dbl)
      n248 = Add(x=w53, y=w54) -> (x+y=w111:dbl)
      n249 = Build Array(w128, w127, w133, w132, w131, w130, w129, w126) -> (w125:dbl[])
      n250 = local read "Reset Data Acquisition\nAnd UI Updating"() -> (w178:bool)
      n251 = Build Array(w110, w110, w114, w114, w110) -> (w106:dbl[])
      n252 = Build Array(w111, w112, w112, w111, w111) -> (w107:dbl[])
      n253 = Decrement(x="LeftSignalA") -> (x-1=w95:dbl)
      n254 = Decrement(x="LefftSignalB") -> (x-1=w97:dbl)
      n255 = Decrement(x="RightSignalB") -> (x-1=w93:dbl)
      n256 = Decrement(x="RightSignalA") -> (x-1=w91:dbl)
      n257 = local read "PointCluster"() -> (w103:cluster{dbl[], dbl[]})
      n258 = Bundle(w106, w107) -> (w113:cluster{dbl[], dbl[]})  [unwired: 1 in]
      n259 = local read "trialFilteredData"() -> (→"Trial Raw Waveforms":waveform(dbl)[])
      n260 = Index Array(array=w125, index=w95) -> (element=w102:dbl)
      n261 = Index Array(array=w125, index=w97) -> (element=w101:dbl)
      n262 = Index Array(array=w125, index=w93) -> (element=w123:dbl)
      n263 = Index Array(array=w125, index=w91) -> (element=w124:dbl)
      n264 = Add(x=w102, y=w101) -> (x+y=w100:dbl)
      n265 = Add(x=w124, y=w123) -> (x+y=w121:dbl)
      n266 = Divide(x=w100, y=2.0) -> (x/y=w68:dbl)
      "RMS Left" <- w68
      "LeftMovingAvg" <- w68
      n267 = Build Array(w103, w113) -> (→"2d target":cluster{dbl[], dbl[]}[])
      n268 = Divide(x=w121, y=2.0) -> (x/y=w69:dbl)
      "RMS Right" <- w69
      "RightMovingAvg" <- w69
      n269 = Add(x=w68, y=w69) -> (x+y=w119:dbl)
      n270 = Divide(x=w119, y=2.0) -> (x/y=w117:dbl)
      n271 = local write "combined y value"(w117) -> ()
    }
    n272 = local write "Reset Data Acquisition\nAnd UI Updating"("End Program") -> ()
    "Bufffer Index" <- 0.0 ("Bufffer Index")
  }
  "Trial In Progress" <- FALSE ("Trial In Progress")
  "Acquiring Max" <- FALSE ("Acquiring Max")
